vi "ReadPathIniKey.vi"(7 "Section":string, 8 "error in (no error)":errorcluster, 10 "Key":string, 11 "refnum In":T1) -> (0 "error out":errorcluster, 2 "Value":path, 3 "refnum out":T1)   [LabVIEW 2013]
uses:
  <vilib>/Utility/config.llb/Config Data RefNum.ctl
  090 - ERRORS/Ctrls/EnumErrors.ctl
  <vilib>/Utility/config.llb/Read Key (Path).vi
  <vilib>/Utility/config.llb/NI_LVConfig.lvlib
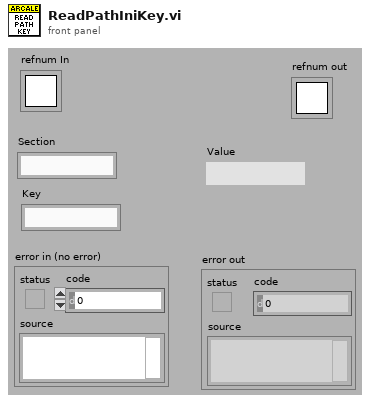
[diagram p1: front panel]
types:
  T1 = typedef "NI_LVConfig.lvlib/Config Data RefNum.ctl" = refnum<k1>
  T2 = typedef "EnumErrors.ctl" = enum16{"VI non trouvé !", "Clé non trouvée", "Timeout", "Le VI tourne déjà", "Erreur de séparateur décimal", "Référence non trouvée"}
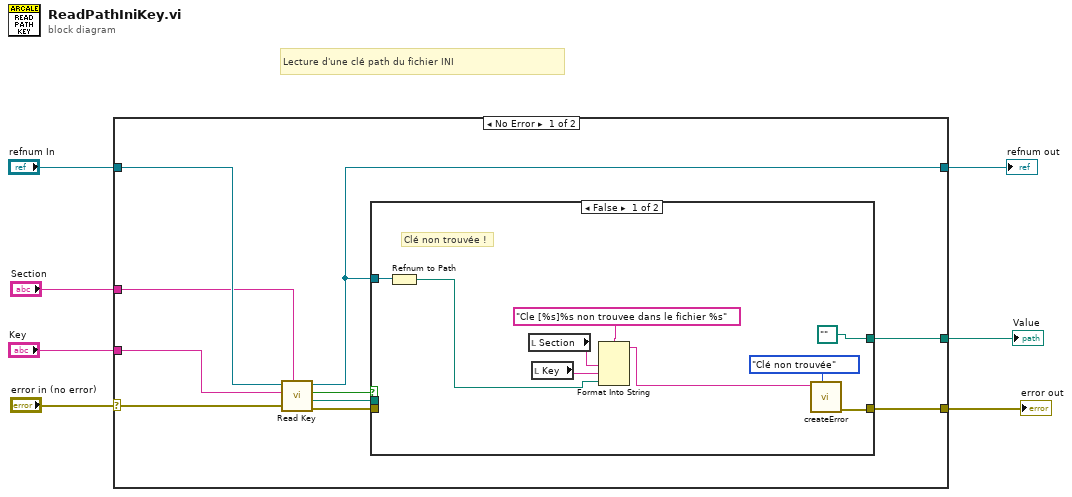
[diagram p0: block diagram]
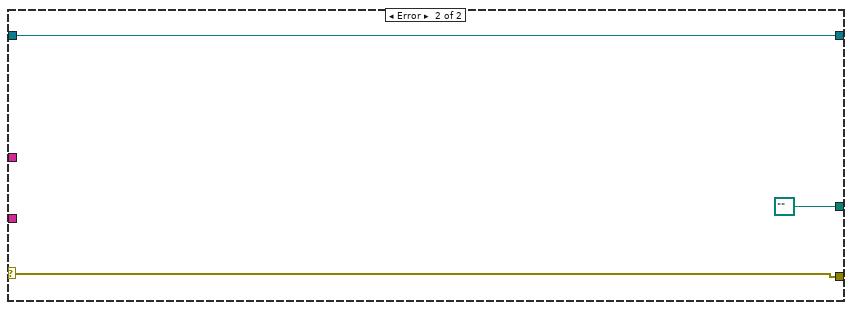
[diagram p3: hidden frame]
diagram:
  # "Lecture d'une clé path du fichier INI"
  n1 = case shown="No Error" "error in (no error)" {
    selector: "error in (no error)" -> [w17 w31]
    tunnel: "refnum In" -> [w16 w30]
    tunnel: "Section" -> [w15 _]
    tunnel: "Key" -> [w14 _]
    tunnel: [w8 w30] -> w3
    tunnel: [w10 path "" ("Valeur")] -> w2
    tunnel: [w9 w31] -> w1
    frame No Error {
      n2 = call-poly <vilib>:"Read Key.vi"("section"=w15, "error in (no error)"=w17, "key"=w14, "refnum"=w16) -> ("error out"=w12:errorcluster, "value"=w11:path, "found?"=w13:bool, "refnum out"=w8:T1)  [unwired: 2 in, 2 out]
      n3 = case shown="False" w13 {
        tunnel: w12 -> [_ w28]
        tunnel: w11 -> [_ w27]
        tunnel: [path "" ("Valeur") w27] -> w10
        tunnel: [w23 w28] -> w9
        tunnel: w8 -> [w21 _]
        frame False {
          # "Clé non trouvée !"
          n4 = Refnum to Path(1:w21) -> (0:w20:path)
          n5 = local read "Section"() -> (w25:string)
          n6 = local read "Key"() -> (w24:string)
          n7 = Format Into String(format string="Cle [%s]%s non trouvee dans le fichier %s", w25, w24, w20) -> (resulting string=w22:string)  [unwired: 2 in, 1 out]
          n8 = call "createError.vi"("ErrorCode"=EnumErrors."Clé non trouvée", "message"=w22) -> ("error out"=w23:errorcluster)  [unwired: 2 in, 7 out]
        }
        frame True {
          # "Clé trouvée !!!"
        }
      }
    }
    frame Error {
    }
  }
  "error out" <- w1
  "refnum out" <- w3
  "Value" <- w2
